vi "Kodu.vi"() -> ()   [LabVIEW 2018]
panel:
  in  "Stop":bool
  in  "length (rest) 2":i32
  in  "offset (0) 2":i32
  in  "length (rest)":i32
  in  "offset (0)":i32
  out "substring 2":string
  out "substring":string
  out "text":string
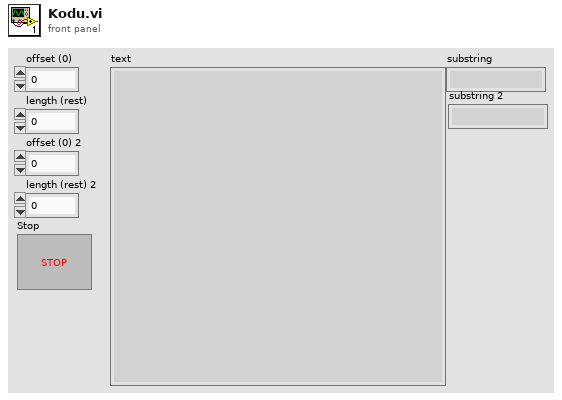
[diagram p1: front panel]
types:
  T1 = enum16{"open", "replace", "create", "open or create", "replace or create", "replace or create with confirmation"}
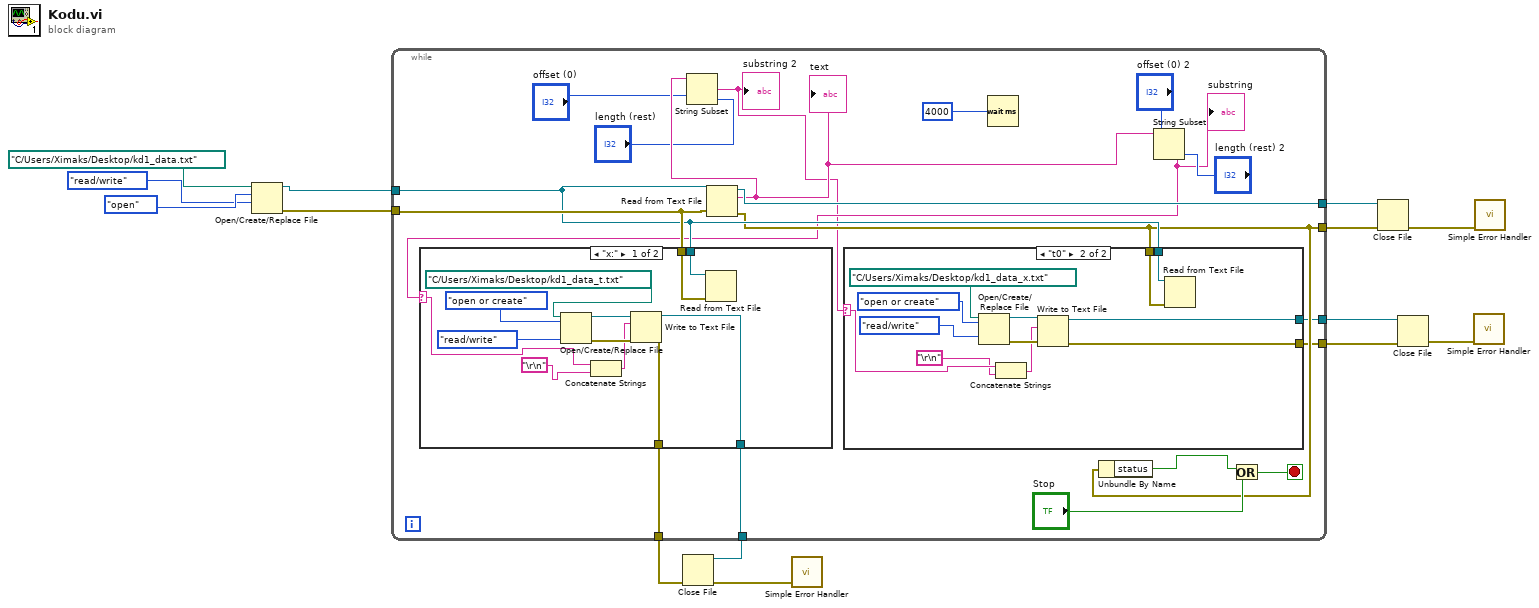
[diagram p0: block diagram]
diagram:
  n1 = Open/Create/Replace File(file path (use dialog)=path "C:/Users/Ximaks/Desktop/kd1_data.txt", operation (0:open)=T1."open", access (0:read/write)=enum16{"read/write", "read-only", "write-only"}."read/write") -> (refnum out=w7:refnum<file>, error out=w8:errorcluster)  [unwired: 3 in, 1 out]
  n2 = while {
    tunnel: [w33] -> w10
    tunnel: [w22] -> w9
    tunnel: w8 -> [w27]
    tunnel: w7 -> [w26]
    tunnel: [w21] -> w6
    tunnel: [w20] -> w5
    tunnel: [w19] -> w2
    tunnel: [w18] -> w1
    stop <- w25 stop-if-true
    n3 = Read from Text File(file (use dialog)=w26, error in=w27) -> (refnum out=w33:refnum<file>, text=w32:string, error out=w22:errorcluster)  [unwired: 2 in, 1 out]
    "text" <- w32
    n4 = String Subset(string=w32, offset (0)="offset (0)", length (rest)="length (rest)") -> (substring=w15:string)
    "substring 2" <- w15
    n5 = case shown="\"t0\"" w15 {
      selector: w15 -> [_ w39]
      tunnel: w26 -> [w34 w47]
      tunnel: w22 -> [w35 w46]
      tunnel: [w34 w38] -> w21
      tunnel: [w35 w37] -> w20
      frame "", Default {
      }
      frame "t0" {
        n6 = Open/Create/Replace File(file path (use dialog)=path "C:/Users/Ximaks/Desktop/kd1_data_x.txt", operation (0:open)=T1."open or create", access (0:read/write)=enum16{"read/write", "read-only", "write-only"}."read/write") -> (refnum out=w44:refnum<file>, error out=w45:errorcluster)  [unwired: 3 in, 1 out]
        n7 = Concatenate Strings(w39, "\r\n") -> (w40:string)
        n8 = Write to Text File(file (use dialog)=w44, text=w40, error in=w45) -> (refnum out=w38:refnum<file>, error out=w37:errorcluster)  [unwired: 1 in, 1 out]
        n9 = Read from Text File(file (use dialog)=w47, error in=w46) -> ()  [unwired: 2 in, 4 out]
      }
    }
    n10 = Wait (ms)(milliseconds to wait=4000) -> ()  [unwired: 1 out]
    n11 = Unbundle By Name(w22) -> ("status"=w24:bool)
    n12 = String Subset(string=w32, offset (0)="offset (0) 2", length (rest)="length (rest) 2") -> (substring=w16:string)
    "substring" <- w16
    n13 = case shown="\"x:\"" w16 {
      selector: w16 -> [w51 _]
      tunnel: w26 -> [w59 w60]
      tunnel: w27 -> [w58 w61]
      tunnel: [w50 w60] -> w19
      tunnel: [w49 w61] -> w18
      frame "x:" {
        n14 = Open/Create/Replace File(file path (use dialog)=path "C:/Users/Ximaks/Desktop/kd1_data_t.txt", operation (0:open)=T1."open or create", access (0:read/write)=enum16{"read/write", "read-only", "write-only"}."read/write") -> (refnum out=w57:refnum<file>, error out=w56:errorcluster)  [unwired: 3 in, 1 out]
        n15 = Concatenate Strings(w51, "\r\n") -> (w52:string)
        n16 = Write to Text File(file (use dialog)=w57, text=w52, error in=w56) -> (refnum out=w50:refnum<file>, error out=w49:errorcluster)  [unwired: 1 in, 1 out]
        n17 = Read from Text File(file (use dialog)=w59, error in=w58) -> ()  [unwired: 2 in, 4 out]
      }
      frame "", Default {
      }
    }
    n18 = Or(x=w24, y="Stop") -> (x .or. y?=w25:bool)
  }
  n19 = Close File(refnum=w2, error in=w1) -> (error out=w3:errorcluster)  [unwired: 1 out]
  n20 = call <vilib>:"Simple Error Handler.vi"("error in (no error)"=w3) -> ()  [unwired: 4 in, 5 out]
  n21 = Close File(refnum=w10, error in=w9) -> (error out=w11:errorcluster)  [unwired: 1 out]
  n22 = Close File(refnum=w6, error in=w5) -> (error out=w4:errorcluster)  [unwired: 1 out]
  n23 = call <vilib>:"Simple Error Handler.vi"("error in (no error)"=w4) -> ()  [unwired: 4 in, 5 out]
  n24 = call <vilib>:"Simple Error Handler.vi"("error in (no error)"=w11) -> ()  [unwired: 4 in, 5 out]
